vi "H5Ldelete_by_idx.vi"(5 "Order":T1 items=["H5_ITER_UNKNOWN"=-1, "H5_ITER_INC"=0, "H5_ITER_DEC"=1], 6 "lapl_id":T3, 7 "Index Field":T2 items=["H5_INDEX_UNKNOWN"=-1, "H5_INDEX_NAME"=0, "H5_INDEX_CRT_ORDER"=1], 8 "error in (no error)":errorcluster, 9 "Index":u64, 10 "Group Name":string=".", 11 "Location Ref":T3) -> (0 "error out":errorcluster, 3 "Location Ref out":T3)   [LabVIEW 2017]
doc: "Removes the nth link in a group."
uses:
  <vilib>/UPVI/lvhdf5/library.llb/HDF5 Ref.ctl
  <vilib>/UPVI/lvhdf5/library.llb/H5_index_t.ctl
  <vilib>/UPVI/lvhdf5/library.llb/H5_iter_order_t.ctl
  <vilib>/UPVI/lvhdf5/hdf5.dll
panel:
  # "LVHDF5 Toolkit\nCopyright (c) 2005-2013 by Jason D. Sommerville\nCopyright (c) 2014-2015 by UPVI, LLC.\n\nThis use and distribution of this file is governed by the terms found in \nLICENSE.txt distributed with this toolkit and installed at\n <user.lib>\\_lvhdf5\\LICENSE.txt"
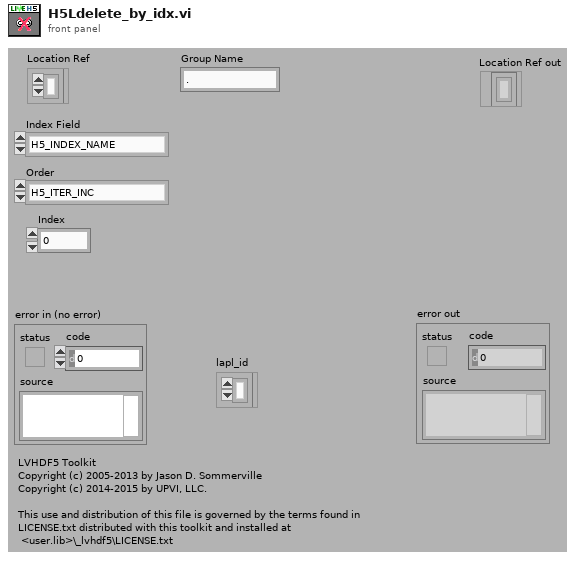
[diagram p1: front panel]
types:
  T1 = typedef "H5_iter_order_t.ctl" = i32
  T2 = typedef "H5_index_t.ctl" = i32
  T3 = typedef "HDF5 Ref.ctl" = refnum<k1>
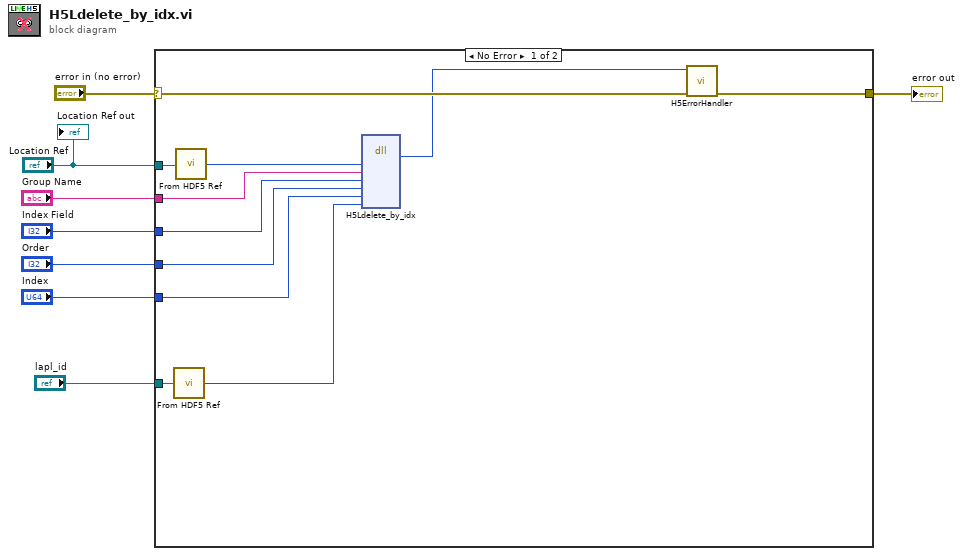
[diagram p0: block diagram]
diagram:
  n1 = case shown="No Error" "error in (no error)" {
    selector: "error in (no error)" -> [w19 w20]
    tunnel: [w18 w20] -> w7
    tunnel: "lapl_id" -> [w17 _]
    tunnel: "Location Ref" -> [w14 _]
    tunnel: "Group Name" -> [w12 _]
    tunnel: "Index Field" -> [w11 _]
    tunnel: "Order" -> [w10 _]
    tunnel: "Index" -> [w9 _]
    frame No Error {
      n2 = call <vilib>:"From HDF5 Ref.vi"("HDF5 Ref"=w17) -> ("I32"=w16:i32)
      n3 = call <vilib>:"From HDF5 Ref.vi"("HDF5 Ref"=w14) -> ("I32"=w13:i32)
      n4 = dll-call lib="C:/Program Files/National Instruments/LabVIEW 2017/vi.lib/UPVI/lvhdf5/hdf5.dll" fn="H5Ldelete_by_idx"("loc_id"=w13, "group_name"=w12, "index_field"=w11, "order"=w10, "n"=w9, "lapl_id"=w16) -> ("return type"=w15:i32)  [unwired: 9 in, 2 out]
      n5 = call <vilib>:"H5ErrorHandler.vi"("error in (no error)"=w19, "herr_t"=w15) -> ("error out"=w18:errorcluster)  [unwired: 3 in, 4 out]
    }
    frame Error {
    }
  }
  "error out" <- w7
  "Location Ref out" <- "Location Ref"
